vi "Untitled 2.vi"() -> ()   [LabVIEW 2016]
panel:
  in  "Calc area":bool
  out "Array":waveform(dbl)[](array[waveform])
  in  "hide chart":bool
  in  "stop graph":bool
  out "Waveform Chart":u32(graph)
  out "main Graph 2":waveform(dbl)[](graph)
  out "XY Graph":cluster{dbl[], dbl[]}[](graph)
  out "graph loop time":u32
  out "main Graph":T1(graph)={"heat_LastData[0]"=21.230000000000018, "heat_LastData[1]"=-273.15, "heat_LastData[2]"=0.0, "heat_LastData[3]"=0.0, "heat_LastData[4]"=0.0, "heat_LastData[5]"=0.0, "heat_LastData[6]"=0.0, "heat_LastData[7]"=0.0, "heat_LastData[8]"=0.0}
  out "RGA_LastData":sgl[](array[numeric]) format="%.2e"
  in  "stop":bool
  out "heat_LastData":dbl[](array[numeric])
  in  "number of materials":dbl
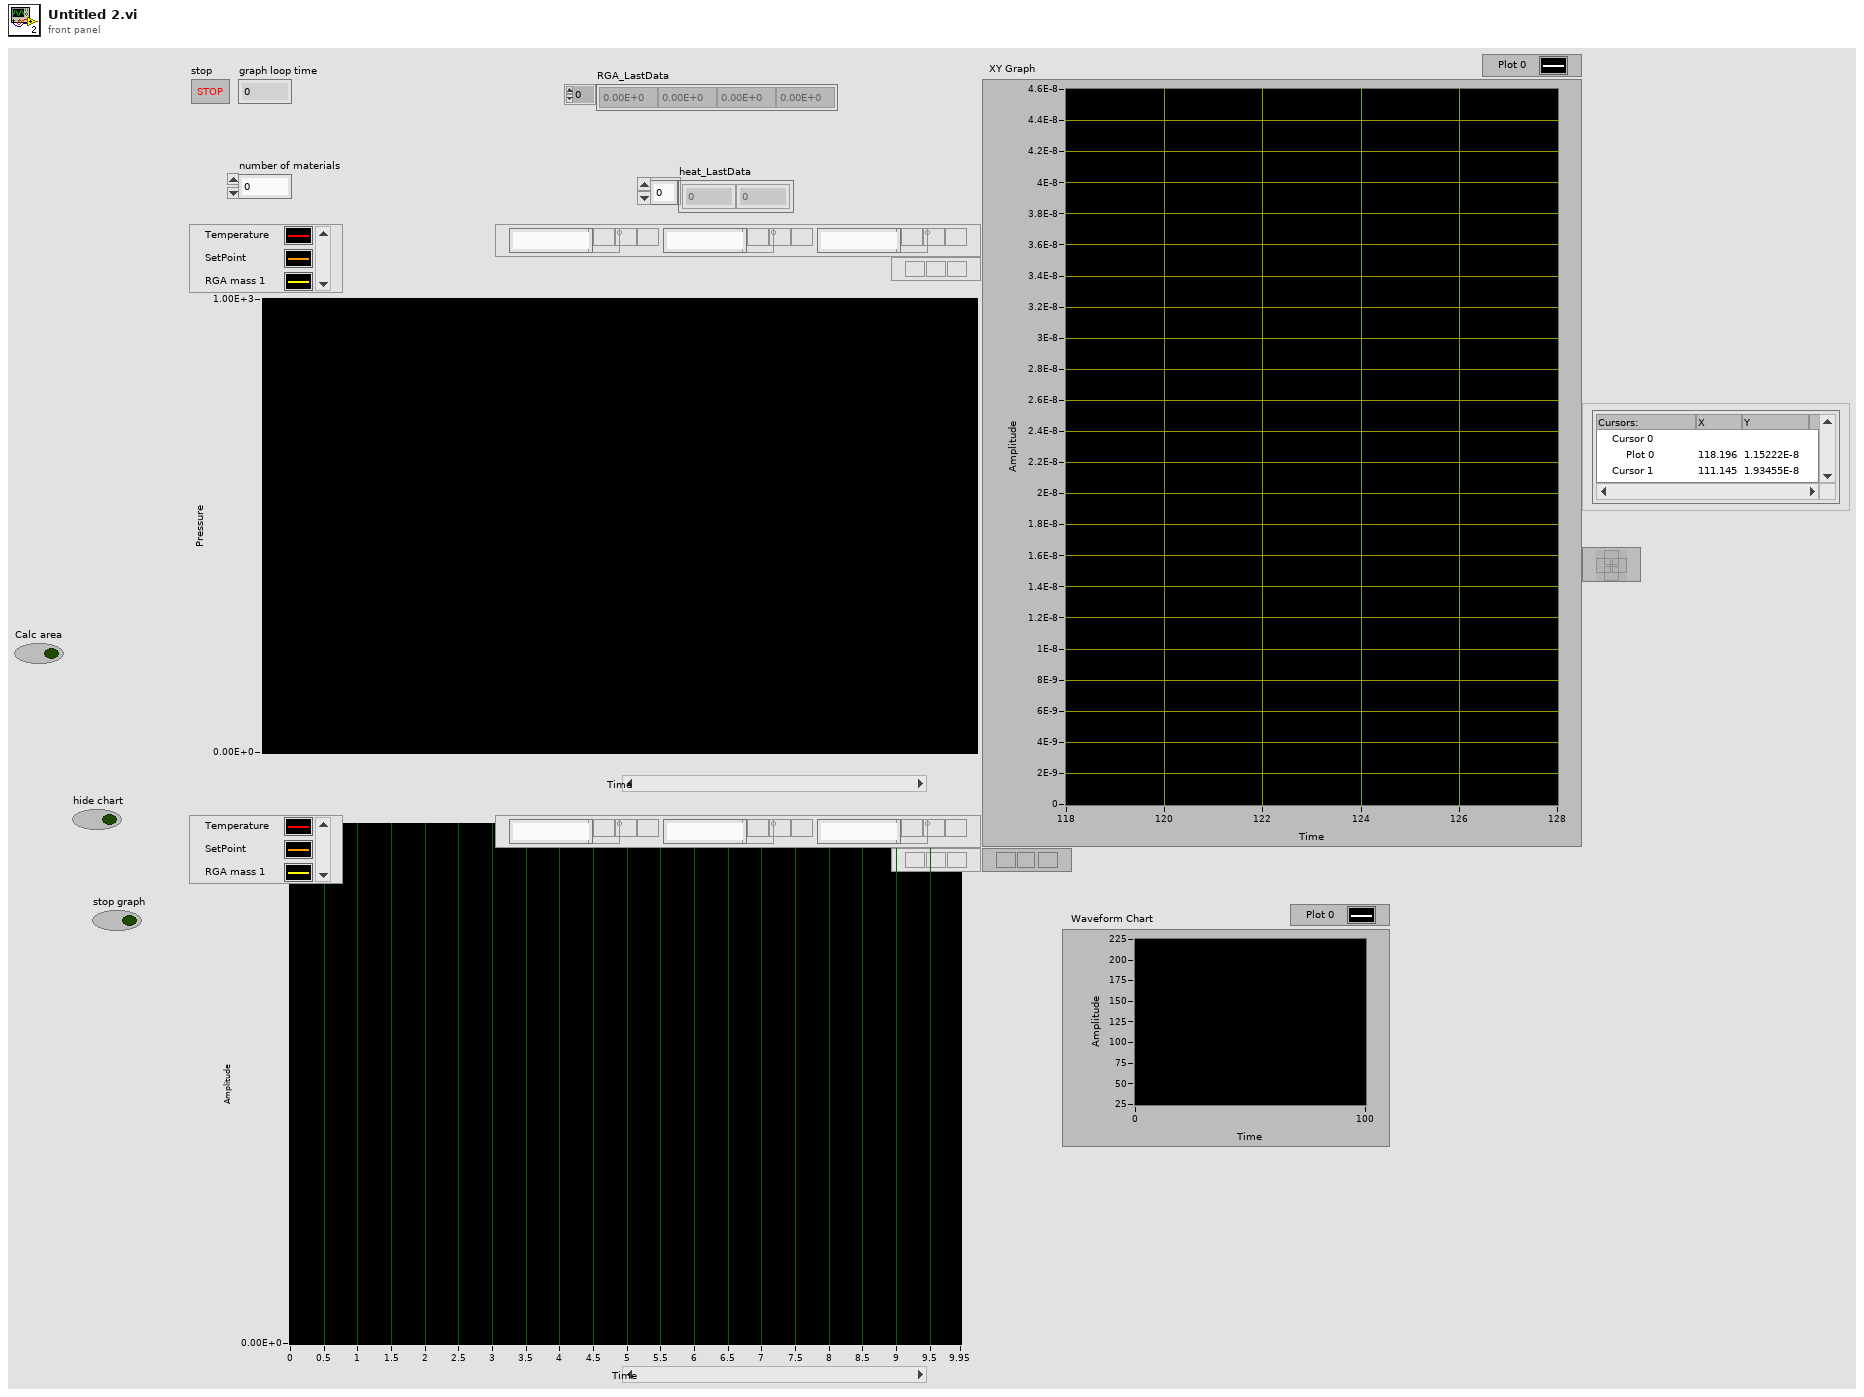
[diagram p1: front panel]
types:
  T1 = cluster{"heat_LastData[0]":dbl, "heat_LastData[1]":dbl, "heat_LastData[2]":dbl, "heat_LastData[3]":dbl, "heat_LastData[4]":dbl, "heat_LastData[5]":dbl, "heat_LastData[6]":dbl, "heat_LastData[7]":dbl, "heat_LastData[8]":dbl}
  T2 = cluster{"heat_LastData[0]":dbl, "heat_LastData[1]":dbl, "heat_LastData[2]":dbl, "heat_LastData[3]":dbl, "heat_LastData[4]":dbl, "heat_LastData[5]":dbl, "heat_LastData[6]":dbl, "heat_LastData[7]":dbl, "heat_LastData[8]":dbl}[]
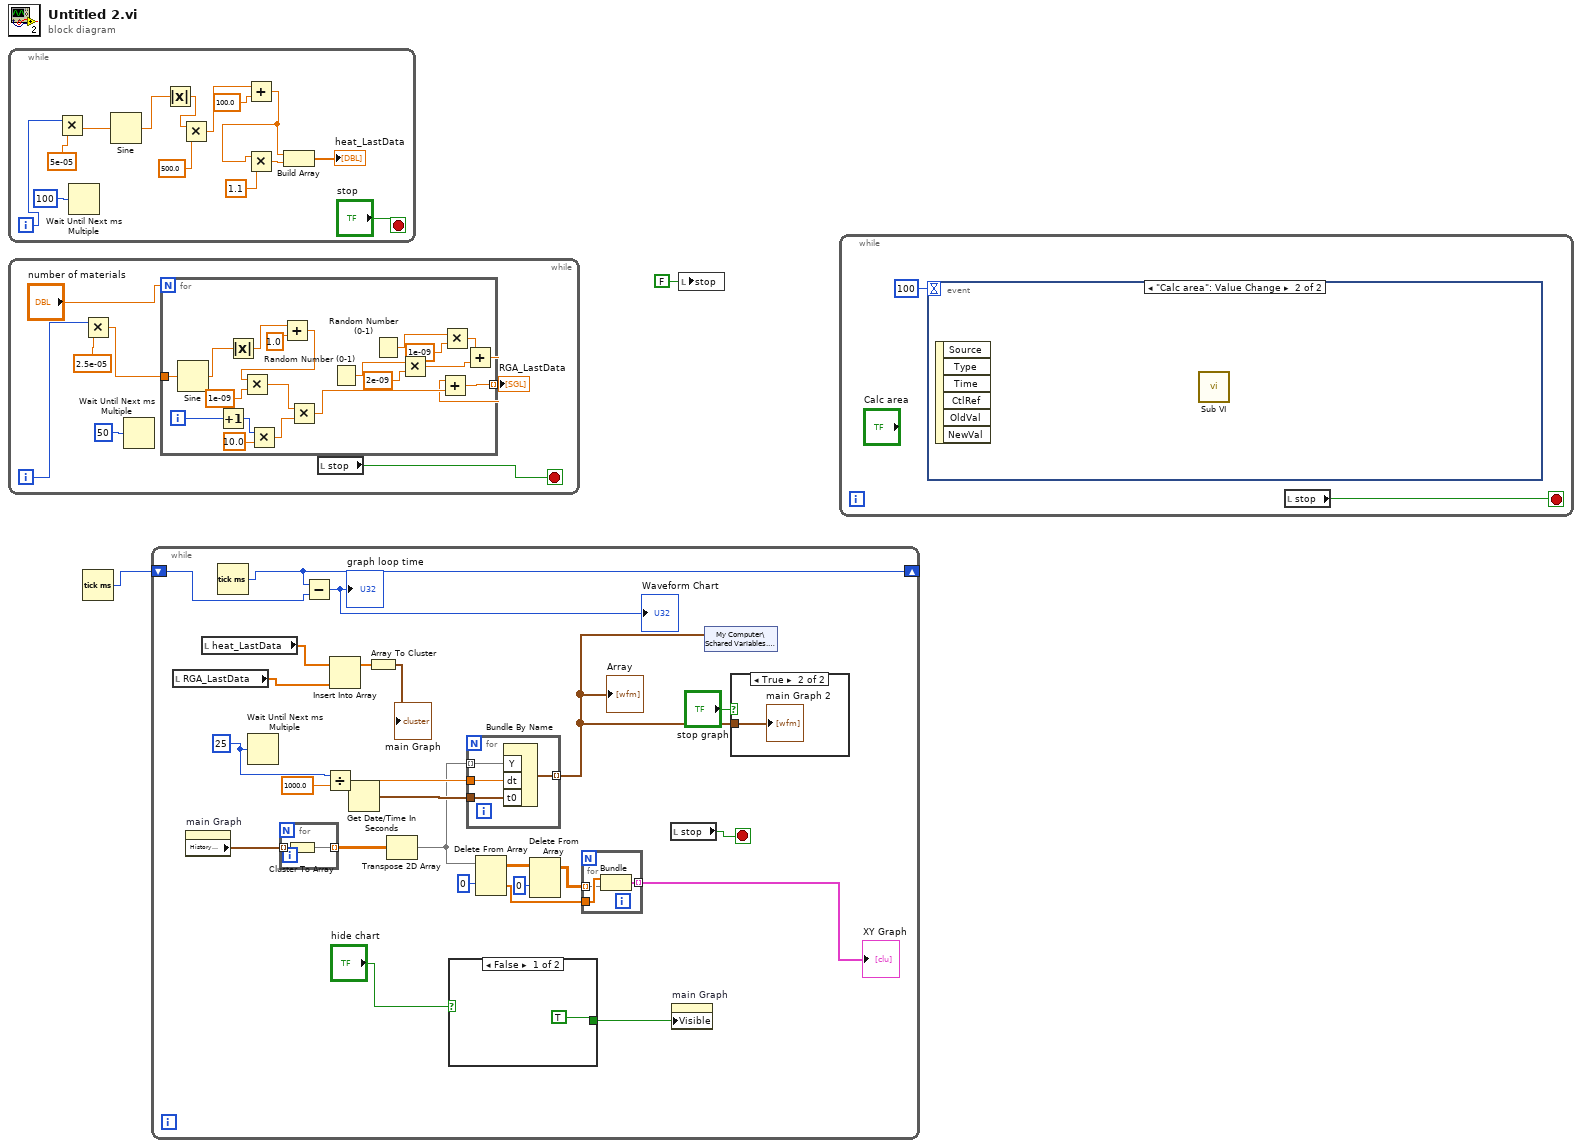
[diagram p0: block diagram]
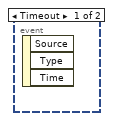
[diagram p2: hidden frame]
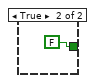
[diagram p3: hidden frame]
diagram:
  n1 = while {
    i -> [w15]
    stop <- "stop" stop-if-true
    n2 = Multiply(x=w15, y=5e-05) -> (x*y=w13:dbl)
    n3 = Wait Until Next ms Multiple(millisecond multiple=u32 100) -> ()  [unwired: 1 out]
    n4 = Sine(x=w13) -> (sin(x)=w8:dbl)
    n5 = Absolute Value(x=w8) -> (abs(x)=w7:dbl)
    n6 = Multiply(x=w7, y=500.0) -> (x*y=w5:dbl)
    n7 = Add(x=w5, y=100.0) -> (x+y=w3:dbl)
    n8 = Multiply(x=w3, y=1.1) -> (x*y=w10:dbl)
    n9 = Build Array(w3, w10) -> (→"heat_LastData":dbl[])
  }
  n10 = while {
    i -> [w20]
    stop <- w23 stop-if-true
    n11 = Multiply(x=w20, y=2.5e-05) -> (x*y=w19:dbl)
    n12 = Wait Until Next ms Multiple(millisecond multiple=u32 50) -> ()  [unwired: 1 out]
    n13 = for {
      N: "number of materials" -> [_]
      tunnel: w19 -> [w36]
      tunnel: [w32] -> w17 mode=indexing
      i -> [w41]
      n14 = Sine(x=w36) -> (sin(x)=w40:dbl)
      n15 = Increment(x=w41) -> (x+1=w25:i32)
      n16 = Absolute Value(x=w40) -> (abs(x)=w38:dbl)
      n17 = Multiply(x=w25, y=10.0) -> (x*y=w24:dbl)
      n18 = Add(x=w38, y=1.0) -> (x+y=w37:dbl)
      n19 = Multiply(x=w37, y=1e-09) -> (x*y=w42:dbl)
      n20 = Multiply(x=w42, y=w24) -> (x*y=w33:dbl)
      n21 = Random Number (0-1)() -> (number: 0 to 1=w30:dbl)
      n22 = Random Number (0-1)() -> (number: 0 to 1=w34:dbl)
      n23 = Multiply(x=w30, y=2e-09) -> (x*y=w28:dbl)
      n24 = Multiply(x=w34, y=1e-09) -> (x*y=w29:dbl)
      n25 = Add(x=w29, y=w28) -> (x+y=w27:dbl)
      n26 = Add(x=w27, y=w33) -> (x+y=w32:dbl)
    }
    "RGA_LastData" <- w17
    n27 = local read "stop"() -> (w23:bool)
  }
  n28 = Tick Count (ms)() -> (millisecond timer value=w1:u32)
  n29 = while {
    shift-right: [w65] -> _
    shift-left: w1 -> [w64]
    stop <- w66 stop-if-true
    w53 = u32 25 ("millisecond multiple")
    n30 = local read "RGA_LastData"() -> (w67:sgl[])
    n31 = property on="main Graph" class="WFChart (strict)"() -> ("History Data"=w57:T2)  [unwired: 2 in, 2 out]
    n32 = local read "heat_LastData"() -> (w68:dbl[])
    n33 = Tick Count (ms)() -> (millisecond timer value=w65:u32)
    n34 = Wait Until Next ms Multiple(millisecond multiple=w53) -> ()  [unwired: 1 out]
    n35 = for {
      tunnel: w57 -> [w80] mode=indexing
      tunnel: [w79] -> w52 mode=indexing
      n36 = Cluster To Array(cluster=w80) -> (array=w79:dbl[])
    }
    n37 = Subtract(x=w65, y=w64) -> (x-y=→"graph loop time" →"Waveform Chart":u32)
    n38 = Divide(x=w53, y=1000.0) -> (x/y=w54:dbl)
    n39 = Insert Into Array(array=w68, new element=w67) -> (w44:dbl[])  [unwired: 1 in]
    n40 = Get Date/Time In Seconds() -> (seconds since 1Jan1904=w56:timestamp)
    n41 = Array To Cluster(array=w44) -> (cluster=→"main Graph":T1)
    n42 = Transpose 2D Array(2D array=w52) -> (transposed array=w51:dbl[][])
    n43 = case shown="False" "hide chart" {
      tunnel: [TRUE ("Visible") FALSE ("Visible")] -> w47
      frame False {
      }
      frame True {
      }
    }
    n44 = for {
      tunnel: w56 -> [w75]
      tunnel: w54 -> [w74]
      tunnel: w51 -> [w73] mode=indexing
      tunnel: [w72] -> w45 mode=indexing
      n45 = Bundle By Name("Y"=w73, "dt"=w74, "t0"=w75) -> (w72:waveform(dbl))  [unwired: 1 out]
    }
    "Array" <- w45
    n46 = Delete From Array(array=w51, index (row)=0) -> (deleted portion=w60:dbl[], array with subset deleted=w62:dbl[][])  [unwired: 2 in]
    n47 = Delete From Array(array=w62, index (row)=0) -> (array with subset deleted=w58:dbl[][])  [unwired: 2 in, 1 out]
    n48 = for {
      tunnel: w58 -> [w77] mode=indexing
      tunnel: w60 -> [w78]
      tunnel: [w76] -> w59 mode=indexing
      n49 = Bundle(w78, w77) -> (w76:cluster{dbl[], dbl[]})  [unwired: 1 in]
    }
    "XY Graph" <- w59
    n50 = local read "stop"() -> (w66:bool)
    n51 = property on="main Graph" class="WFChart (strict)"("Visible"=w47) -> ()  [unwired: 2 in, 2 out]
    n52 = shared-variable "My Computer\\Schared Variables.lvlib\\Array"(w45) -> ()  [unwired: 1 in, 1 out]
    n53 = case shown="True" "stop graph" {
      tunnel: w45 -> [_ w71]
      frame False {
      }
      frame True {
        "main Graph 2" <- w71
      }
    }
  }
  n54 = local write "stop"(FALSE ("stop")) -> ()
  n55 = while {
    stop <- w81 stop-if-true
    n56 = event shown="[1] \"Calc area\": Value Change" {
      selector: _ -> [_ _]
      dyn-events: _ -> [_ _]
      timeout: 100 -> [_ _]
      event Timeout {
        n57 = event-data() -> ()  [unwired: 1 in, 3 out]
      }
      event "Calc area": Value Change {
        n58 = event-data() -> ()  [unwired: 1 in, 6 out]
        n59 = call "Sub VI.vi"() -> ()  [unwired: 12 in]
      }
    }
    n60 = local read "stop"() -> (w81:bool)
  }
